vi "Begin.vi"(8 "error in":errorcluster) -> (0 "error out":errorcluster)   [LabVIEW 2019]
doc: "Called before other user functions, this VI is expected to open initial I/O refnums, load in file data, and do all program initialization. Notice that the <B>error out</B> terminal is simply used for data flow. Wiring it to other structures or subVIs ensures that this VI runs first."
uses:
  <vilib>/Rock Robotics/SystemInterfaces/i2clib/i2c_bus.ctl
  <vilib>/Rock Robotics/WPI/DriverStation/WPI_DriverStationRobotMode2.ctl
  <vilib>/Rock Robotics/WPI/Joystick/WPI_JoystickDeviceEnum.ctl
  <vilib>/Rock Robotics/WPI/SafetyOutput/WPI_SafetyOutputConfigMenu.ctl
  <vilib>/Rock Robotics/WPI/ThirdParty/Phoenix-LabVIEW/Motor Controller/Controls/CTRE_Phoenix_MotorControl_FeedbackDevice.ctl
  <vilib>/Rock Robotics/WPI/Solenoid/WPI_SolenoidChannel.ctl
  <vilib>/Rock Robotics/WPI/ThirdParty/Phoenix-LabVIEW/Motor Controller/Controls/CTRE_Phoenix_MotorControl_ControlMode.ctl
  <vilib>/Rock Robotics/WPI/ThirdParty/Phoenix-LabVIEW/Motor Controller/Controls/CTRE_Phoenix_MotorControl_FeedbackDevice_TalonFX.ctl
  <vilib>/Rock Robotics/WPI/ThirdParty/Phoenix-LabVIEW/Motor Controller/Controls/CTRE_Phoenix_MotorControl_NeutralMode.ctl
  <vilib>/Rock Robotics/WPI/ThirdParty/REV Robotics/SPARK MAX/Typedef/Spark MAX Motor Type.ctl
  <vilib>/Rock Robotics/WPI/ThirdParty/Phoenix-LabVIEW/Motor Controller/Controls/CTRE_Phoenix_MotorControl_VelocityMeasurementPeriod.ctl
  <vilib>/Rock Robotics/SystemInterfaces/DIO/FPGA_DIOChannel.ctl
  Robot Global Data.vi
  <vilib>/Rock Robotics/Network Tables/NT Write String Array.vi
  <vilib>/Rock Robotics/WPI/Solenoid/WPI_SolenoidOpenDouble.vi
  <vilib>/Rock Robotics/WPI/RobotDrive/WPI_RobotDriveOpen4MotorWithExistingMotors.vi
panel:
  in  "Blue Calibration":cluster{"R":dbl, "G":dbl, "B":dbl}={"R"=0.143, "G"=0.427, "B"=0.429}
  in  "Green Calibration":cluster{"R":dbl, "G":dbl, "B":dbl}={"R"=0.197, "G"=0.561, "B"=0.24}
  in  "Red Calibration":cluster{"R":dbl, "G":dbl, "B":dbl}={"R"=0.561, "G"=0.323, "B"=0.114}
  in  "Yellow Calibration":cluster{"R":dbl, "G":dbl, "B":dbl}={"R"=0.361, "G"=0.524, "B"=0.113}
  in  "I2C Bus":T1
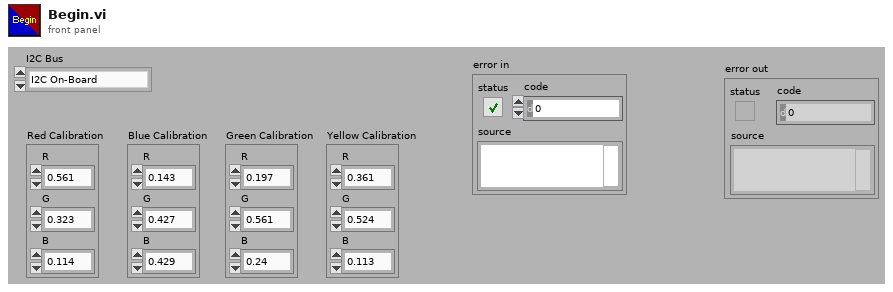
[diagram p1: front panel]
types:
  T1 = typedef "i2c_bus.ctl" = enum16{"I2C On-Board", "I2C MXP", "Invalid"}
  T2 = typedef "WPI_SolenoidChannel.ctl" = enum8{"Solenoid 0", "Solenoid 1", "Solenoid 2", "Solenoid 3", "Solenoid 4", "Solenoid 5", "Solenoid 6", "Solenoid 7", "Invalid"}
  T3 = typedef "FPGA_DIOChannel.ctl" = enum8{"DIO 0", "DIO 1", "DIO 2", "DIO 3", "DIO 4", "DIO 5", "DIO 6", "DIO 7", "DIO 8", "DIO 9", "DIO MXP 0", "DIO MXP 1", "DIO MXP 2", "DIO MXP 3", "DIO MXP 4", "DIO MXP 5", "DIO MXP 6", "DIO MXP 7", "DIO MXP 8", "DIO MXP 9", "DIO MXP 10", "DIO MXP 11", "DIO MXP 12", "DIO MXP 13", "DIO MXP 14", "DIO MXP 15", "SPI Port CS1", "SPI Port CS2", "SPI Port CS3", "SPI Port MISO", "SPI Port MOSI", "Invalid"}
  T4 = typedef "CTRE_Phoenix_MotorControl_VelocityMeasurementPeriod.ctl" = u16
  T5 = typedef "CTRE_Phoenix_MotorControl_NeutralMode.ctl" = enum8{"EEPROMSetting", "Override to Coast", "Override to Brake"}
  T6 = typedef "CTRE_Phoenix_MotorControl_FeedbackDevice_TalonFX.ctl" = i8
  T7 = typedef "CTRE_Phoenix_MotorControl_ControlMode.ctl" = u16
  T8 = typedef "Spark MAX Motor Type.ctl" = enum16{"Brushed", "Brushless"}
  T9 = typedef "CTRE_Phoenix_MotorControl_FeedbackDevice.ctl" = i8
  T10 = typedef "WPI_SafetyOutputConfigMenu.ctl" = enum16{"Enable", "Disable"}
  T11 = typedef "WPI_JoystickDeviceEnum.ctl" = enum16{"USB 0", "USB 1", "USB 2", "USB 3", "USB 4", "USB 5"}
  T12 = typedef "WPI_DriverStationRobotMode2.ctl" = enum16{"Autonomous Disabled", "Autonomous Enabled", "Teleop Disabled", "Teleop Enabled", "Disconnected", "Finish", "Test Disabled", "Test Enabled", "Emergency Stopped"}
  T13 = typedef "Color Sensor V3 DevRef.ctl" = cluster{"I2CDevRef":T14}
  T14 = typedef "WPI_I2CDevRef.ctl" = cluster{"DevStatus":errorcluster, "Device Address":u8, "Handle":i32, "I2C Bus":T1}
  T15 = typedef "WPI_JoystickDevRef.ctl" = cluster{"Device":T11}
  T16 = typedef "WPI_DigitalInputDevRef.ctl" = cluster{"DevStatus":errorcluster, "DIO Channel":T3}
  T17 = typedef "WPI_MotorControlDeviceRef.ctl" = cluster{"DeviceStatus":errorcluster, "Type":T18, "PWM":cluster{"PWM Channel":T19, "DeadBand":T20}, "CAN":cluster{"Device Number":u8, "SetOutput VI Ref":variant, "GetOutput VI Ref":variant, "Enable VI Ref":variant, "Disable VI Ref":variant, "Data":variant}, "Invert":bool, "DIO PWM":cluster{"PWM \"Enable\" Channel":T19, "DIOChannel":T3, "PWM Rate":dbl}}
  T18 = typedef "WPI_MotorControlType.ctl" = enum16{"PWM", "CAN", "DIO PWM"}
  T19 = typedef "FPGA_DIOPWMChannel.ctl" = enum8{"PWM 0", "PWM 1", "PWM 2", "PWM 3", "PWM 4", "PWM 5", "PWM 6", "PWM 7", "PWM 8", "PWM 9", "PWM MXP 0", "PWM MXP 1", "PWM MXP 2", "PWM MXP 3", "PWM MXP 4", "PWM MXP 5", "PWM MXP 6", "PWM MXP 7", "PWM MXP 8", "PWM MXP 9", "Invalid"}
  T20 = typedef "WPI_PWMDeadband.ctl" = cluster{"Name":string, "maxPositivePwm":i32, "minPositivePwm":i32, "centerPwm":i32, "maxNegativePwm":i32, "minNegativePwm":i32, "angularRange":u16}
  T21 = typedef "WPI_SolenoidDevRef.ctl" = cluster{"DevStatus":errorcluster, "Pneumatics Control Module":u8, "Forward Solenoid Channel":T2, "Reverse Solenoid Channel":T2}
  T22 = typedef "WPI_RobotDriveDevRef.ctl" = cluster{"DevStatus":errorcluster, "Motors[]":T17[], "Square Inputs":bool, "Max Output":dbl}
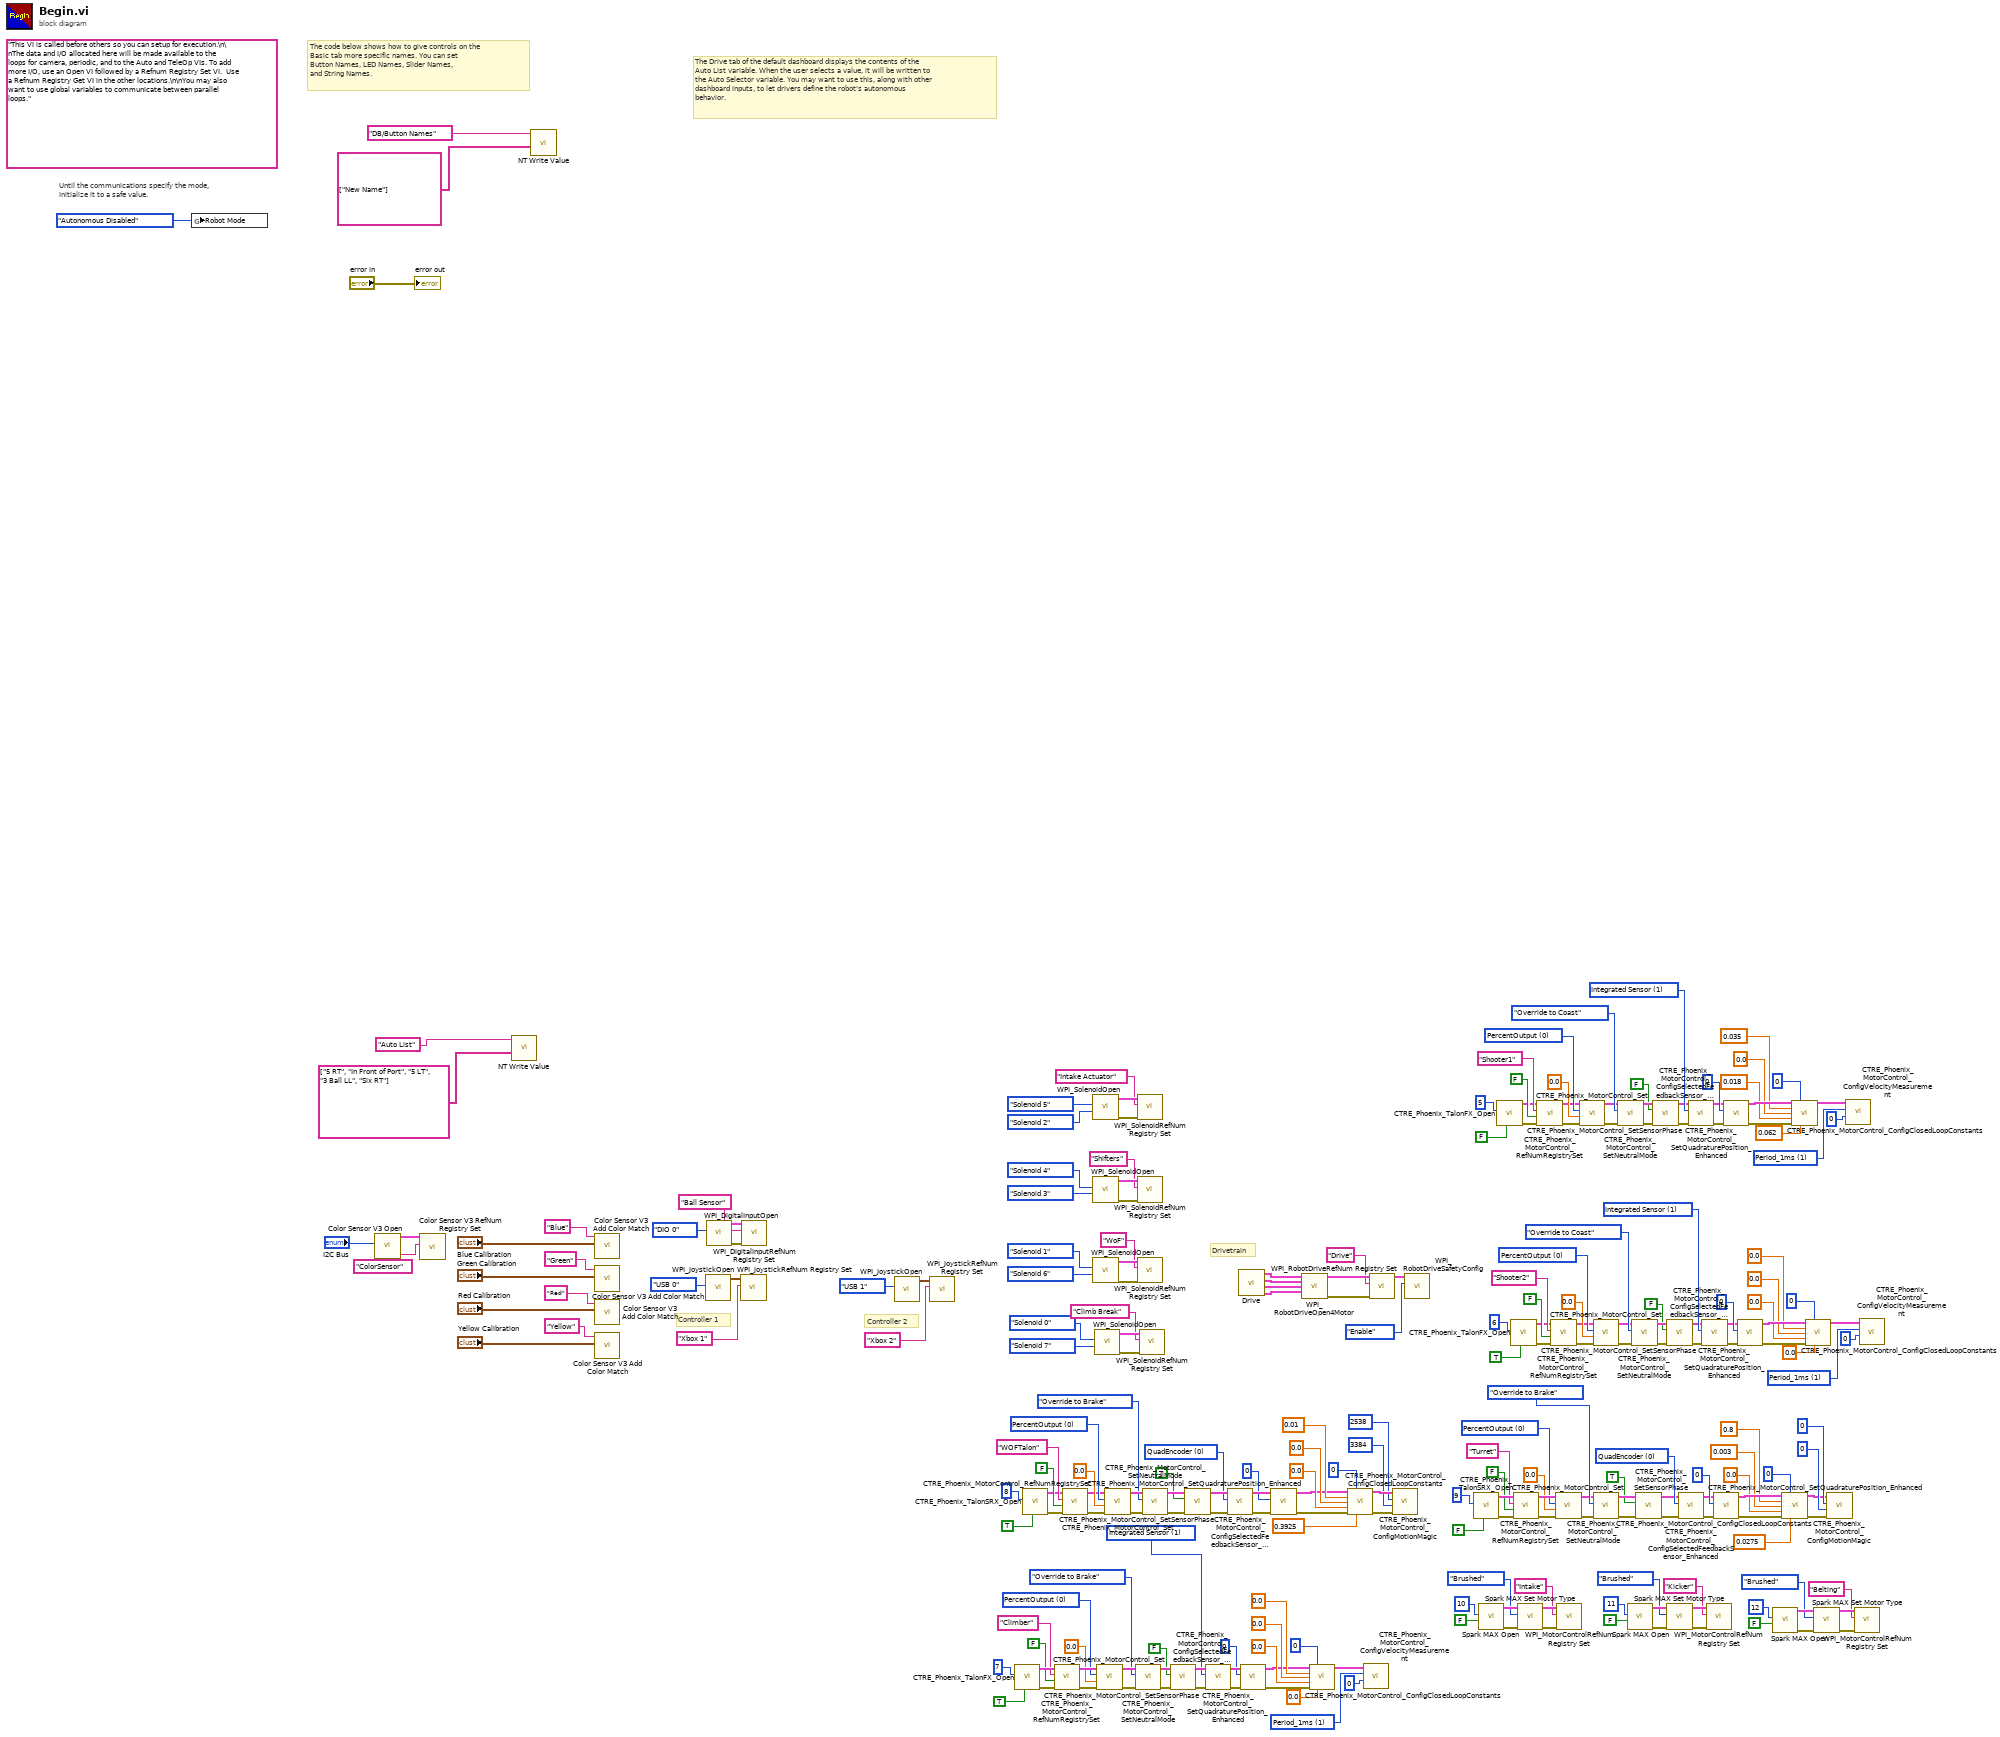
[diagram p0: block diagram]
diagram:
  w21 = T4 1 items=["Period_1ms"=1, "Period_2ms"=2, "Period_5ms"=5, "Period_10ms"=10, "Period_20ms"=20, "Period_25ms"=25, "Period_50ms"=50, "Period_100ms"=100] ("Velocity Measurement Period")
  w82 = T4 1 items=["Period_1ms"=1, "Period_2ms"=2, "Period_5ms"=5, "Period_10ms"=10, "Period_20ms"=20, "Period_25ms"=25, "Period_50ms"=50, "Period_100ms"=100] ("Velocity Measurement Period")
  w66 = T6 1 items=["Integrated Sensor"=1, "Sensor Sum (S0 + S1)"=9, "Sensor Difference (D0 - D1)"=10, "Remote Source 0"=11, "Remote Source 1"=12, "None"=14, "Software Emulated"=15] ("Talon FX Feedback Device")
  w64 = T7 0 items=["PercentOutput"=0, "Position"=1, "Velocity"=2, "Current"=3, "Follower"=5, "MotionProfile"=6, "MotionMagic"=7, "MotionProfileArc"=10, "Disabled"=15] ("Control Mode")
  w47 = T6 1 items=["Integrated Sensor"=1, "Sensor Sum (S0 + S1)"=9, "Sensor Difference (D0 - D1)"=10, "Remote Source 0"=11, "Remote Source 1"=12, "None"=14, "Software Emulated"=15] ("Talon FX Feedback Device")
  w45 = T7 0 items=["PercentOutput"=0, "Position"=1, "Velocity"=2, "Current"=3, "Follower"=5, "MotionProfile"=6, "MotionMagic"=7, "MotionProfileArc"=10, "Disabled"=15] ("Control Mode")
  w128 = T9 0 items=["None"=-1, "QuadEncoder"=0, "Analog"=2, "Tachometer"=4, "Pulse Width Encoded Position"=8, "Sensor Sum (S0 + S1)"=9, "Sensor Difference (D0 - D1)"=10, "Remote Source 0"=11, "Remote Source 1"=12, "Software Emulated"=15] ("Feedback Device")
  w123 = T7 0 items=["PercentOutput"=0, "Position"=1, "Velocity"=2, "Current"=3, "Follower"=5, "MotionProfile"=6, "MotionMagic"=7, "MotionMagicArc"=8, "MotionProfileArc"=10, "Disabled"=15] ("Control Mode")
  w143 = T4 1 items=["Period_1ms"=1, "Period_2ms"=2, "Period_5ms"=5, "Period_10ms"=10, "Period_20ms"=20, "Period_25ms"=25, "Period_50ms"=50, "Period_100ms"=100] ("Velocity Measurement Period")
  w155 = T6 1 items=["Integrated Sensor"=1, "Sensor Sum (S0 + S1)"=9, "Sensor Difference (D0 - D1)"=10, "Remote Source 0"=11, "Remote Source 1"=12, "None"=14, "Software Emulated"=15] ("Talon FX Feedback Device")
  w158 = T7 0 items=["PercentOutput"=0, "Position"=1, "Velocity"=2, "Current"=3, "Follower"=5, "MotionProfile"=6, "MotionMagic"=7, "MotionProfileArc"=10, "Disabled"=15] ("Control Mode")
  w196 = T9 0 items=["None"=-1, "QuadEncoder"=0, "Analog"=2, "Tachometer"=4, "Pulse Width Encoded Position"=8, "Sensor Sum (S0 + S1)"=9, "Sensor Difference (D0 - D1)"=10, "Remote Source 0"=11, "Remote Source 1"=12, "Software Emulated"=15] ("Feedback Device")
  w201 = T7 0 items=["PercentOutput"=0, "Position"=1, "Velocity"=2, "Current"=3, "Follower"=5, "MotionProfile"=6, "MotionMagic"=7, "MotionMagicArc"=8, "MotionProfileArc"=10, "Disabled"=15] ("Control Mode")
  (unwired) "This VI is called before others so you can setup for execution.\n\nThe data and I/O allocated here will be made available to the loops for camera, periodic, and to the Auto and TeleOp VIs. To add more I/O, use an Open VI followed by a Refnum Registry Set VI.  Use a Refnum Registry Get VI in the other locations.\n\nYou may also want to use global variables to communicate between parallel loops."
  # "Controller 2"
  # "Controller 1"
  # "Drivetrain"
  # "The Drive tab of the default dashboard displays the contents of the\nAuto List variable. When the user selects a value, it will be written to\nthe Auto Selector variable. You may want to use this, along with other\ndashboard inputs, to let drivers define the robot's autonomous\nbehavior."
  # "The code below shows how to give controls on the\nBasic tab more specific names. You can set\nButton Names, LED Names, Slider Names,\nand String Names."
  # "Until the communications specify the mode,\ninitialize it to a safe value."
  n1 = global write "Robot Global Data.vi" "Robot Mode"(WPI_DriverStationRobotMode2."Autonomous Disabled" ("Robot Mode")) -> ()
  n2 = call <vilib>:"Color Sensor V3 Open.vi"("I2C Bus"="I2C Bus") -> ("ColorSensorDevRef"=w224:T13)  [unwired: 9 in, 1 out]
  n3 = call <vilib>:"Color Sensor V3 RefNum Registry Set.vi"("refnum name"="ColorSensor", "ColorSensorDevRef"=w224) -> ()  [unwired: 8 in, 2 out]
  n4 = call-poly <vilib>:"NT Write Value.vi"("String Array"=string[] ["5 RT", "In Front of Port", "5 LT", "3 Ball LL", "Six RT"], "Name"="Auto List") -> ()  [unwired: 9 in, 1 out]
  n5 = call-poly <vilib>:"NT Write Value.vi"("String Array"=string[] ["New Name"], "Name"="DB/Button Names") -> ()  [unwired: 9 in, 1 out]
  n6 = call <vilib>:"Color Sensor V3 Add Color Match.vi"("Color"="Blue Calibration", "Name"="Blue") -> ()  [unwired: 10 in]
  n7 = call <vilib>:"Color Sensor V3 Add Color Match.vi"("Color"="Green Calibration", "Name"="Green") -> ()  [unwired: 10 in]
  n8 = call <vilib>:"Color Sensor V3 Add Color Match.vi"("Color"="Red Calibration", "Name"="Red") -> ()  [unwired: 10 in]
  n9 = call <vilib>:"Color Sensor V3 Add Color Match.vi"("Color"="Yellow Calibration", "Name"="Yellow") -> ()  [unwired: 10 in]
  n10 = call <vilib>:"WPI_JoystickOpen.vi"("JoystickDevice"=WPI_JoystickDeviceEnum."USB 0") -> ("JoystickDevRef"=w240:T15)  [unwired: 10 in]
  n11 = call <vilib>:"WPI_DigitalInputOpen.vi"("DIO Channel"=FPGA_DIOChannel."DIO 0") -> ("error out"=w20:errorcluster, "DigitalInputDevRef"=w19:T16)  [unwired: 9 in]
  n12 = call <vilib>:"WPI_JoystickRefNum Registry Set.vi"("refnum name"="Xbox 1", "JoystickDevRef"=w240) -> ()  [unwired: 8 in, 2 out]
  n13 = call <vilib>:"WPI_DigitalInputRefNum Registry Set.vi"("error in (no error)"=w20, "refnum name"="Ball Sensor", "DigitalInputDevRef"=w19) -> ()  [unwired: 7 in, 2 out]
  n14 = call <vilib>:"WPI_JoystickOpen.vi"("JoystickDevice"=WPI_JoystickDeviceEnum."USB 1") -> ("JoystickDevRef"=w221:T15)  [unwired: 10 in]
  n15 = call <vilib>:"WPI_JoystickRefNum Registry Set.vi"("refnum name"="Xbox 2", "JoystickDevRef"=w221) -> ()  [unwired: 8 in, 2 out]
  n16 = call <vilib>:"CTRE_Phoenix_TalonFX_Open.vi"("Invert"=TRUE, "Device Number"=u8 7) -> ("error out"=w173:errorcluster, "CAN Talon SRX Ref"=w172:T17)  [unwired: 8 in]
  n17 = call <vilib>:"CTRE_Phoenix_TalonSRX_Open.vi"("Invert"=TRUE, "Device Number"=u8 8) -> ("error out"=w137:errorcluster, "CAN Talon SRX Ref"=w138:T17)  [unwired: 8 in]
  n18 = call <vilib>:"CTRE_Phoenix_MotorControl_RefNumRegistrySet.vi"("error in (no error)"=w173, "Test Mode Only"=FALSE, "refnum name"="Climber", "PhoenixMotorControlDevRef"=w172) -> ("error out"=w171:errorcluster, "PhoenixMotorControlDevRef"=w170:T17)  [unwired: 6 in]
  n19 = call <vilib>:"CTRE_Phoenix_MotorControl_RefNumRegistrySet.vi"("error in (no error)"=w137, "Test Mode Only"=FALSE, "refnum name"="WOFTalon", "PhoenixMotorControlDevRef"=w138) -> ("error out"=w121:errorcluster, "PhoenixMotorControlDevRef"=w122:T17)  [unwired: 6 in]
  n20 = call-poly <vilib>:"WPI_SolenoidOpen.vi"("Reverse Solenoid Channel"=WPI_SolenoidChannel."Solenoid 2", "Forward Solenoid Channel"=WPI_SolenoidChannel."Solenoid 5") -> ("error out"=w7:errorcluster, "SolenoidDevRef"=w6:T21)  [unwired: 8 in]
  n21 = call-poly <vilib>:"WPI_SolenoidOpen.vi"("Reverse Solenoid Channel"=WPI_SolenoidChannel."Solenoid 3", "Forward Solenoid Channel"=WPI_SolenoidChannel."Solenoid 4") -> ("error out"=w177:errorcluster, "SolenoidDevRef"=w176:T21)  [unwired: 8 in]
  n22 = call-poly <vilib>:"WPI_SolenoidOpen.vi"("Reverse Solenoid Channel"=WPI_SolenoidChannel."Solenoid 6", "Forward Solenoid Channel"=WPI_SolenoidChannel."Solenoid 1") -> ("error out"=w16:errorcluster, "SolenoidDevRef"=w15:T21)  [unwired: 8 in]
  n23 = call-poly <vilib>:"WPI_SolenoidOpen.vi"("Reverse Solenoid Channel"=WPI_SolenoidChannel."Solenoid 7", "Forward Solenoid Channel"=WPI_SolenoidChannel."Solenoid 0") -> ("error out"=w12:errorcluster, "SolenoidDevRef"=w11:T21)  [unwired: 8 in]
  n24 = call <vilib>:"CTRE_Phoenix_MotorControl_Set.vi"("error in (no error)"=w171, "Output"=0.0, "Control Mode"=w158, "PhoenixMotorControlDevRef"=w170) -> ("error out"=w169:errorcluster, "PhoenixMotorControlDevRef"=w168:T17)  [unwired: 6 in]
  n25 = call <vilib>:"CTRE_Phoenix_MotorControl_Set.vi"("error in (no error)"=w121, "Output"=0.0, "Control Mode"=w123, "PhoenixMotorControlDevRef"=w122) -> ("error out"=w132:errorcluster, "PhoenixMotorControlDevRef"=w136:T17)  [unwired: 6 in]
  n26 = call <vilib>:"CTRE_Phoenix_MotorControl_SetNeutralMode.vi"("error in (no error)"=w169, "Motor Control Neutral Mode"=CTRE_Phoenix_MotorControl_NeutralMode."Override to Brake", "PhoenixMotorControlDevRef"=w168) -> ("error out"=w167:errorcluster, "PhoenixMotorControlDevRef"=w166:T17)  [unwired: 7 in]
  n27 = call <vilib>:"WPI_SolenoidRefNum Registry Set.vi"("error in (no error)"=w7, "refnum name"="Intake Actuator", "SolenoidDevRef"=w6) -> ()  [unwired: 7 in, 2 out]
  n28 = call <vilib>:"WPI_SolenoidRefNum Registry Set.vi"("error in (no error)"=w177, "refnum name"="Shifters", "SolenoidDevRef"=w176) -> ()  [unwired: 7 in, 2 out]
  n29 = call <vilib>:"WPI_SolenoidRefNum Registry Set.vi"("error in (no error)"=w16, "refnum name"="WoF", "SolenoidDevRef"=w15) -> ()  [unwired: 7 in, 2 out]
  n30 = call <vilib>:"WPI_SolenoidRefNum Registry Set.vi"("error in (no error)"=w12, "refnum name"="Climb Break", "SolenoidDevRef"=w11) -> ()  [unwired: 7 in, 2 out]
  n31 = call <vilib>:"CTRE_Phoenix_MotorControl_SetNeutralMode.vi"("error in (no error)"=w132, "Motor Control Neutral Mode"=CTRE_Phoenix_MotorControl_NeutralMode."Override to Brake", "PhoenixMotorControlDevRef"=w136) -> ("error out"=w134:errorcluster, "PhoenixMotorControlDevRef"=w133:T17)  [unwired: 7 in]
  n32 = call <vilib>:"CTRE_Phoenix_MotorControl_SetSensorPhase.vi"("error in (no error)"=w167, "PhaseSensor"=FALSE, "PhoenixMotorControlDevRef"=w166) -> ("error out"=w165:errorcluster, "PhoenixMotorControlDevRef"=w164:T17)  [unwired: 7 in]
  n33 = call <vilib>:"CTRE_Phoenix_MotorControl_SetSensorPhase.vi"("error in (no error)"=w134, "PhaseSensor"=TRUE, "PhoenixMotorControlDevRef"=w133) -> ("error out"=w130:errorcluster, "PhoenixMotorControlDevRef"=w129:T17)  [unwired: 7 in]
  n34 = call <vilib>:"CTRE_Phoenix_MotorControl_ConfigSelectedFeedbackSensor_TalonFX.vi"("error in (no error)"=w165, "Talon FX Feedback Device"=w155, "PhoenixMotorControlDevRef"=w164) -> ("error out"=w163:errorcluster, "PhoenixMotorControlDevRef"=w162:T17)  [unwired: 7 in]
  n35 = call <vilib>:"CTRE_Phoenix_MotorControl_ConfigSelectedFeedbackSensor_Enhanced.vi"("error in (no error)"=w130, "Feedback Device"=w128, "PhoenixMotorControlDevRef"=w129) -> ("error out"=w126:errorcluster, "PhoenixMotorControlDevRef"=w127:T17)  [unwired: 7 in]
  n36 = call "Drive.vi"() -> ("Front Right"=w178:T17, "Front Left"=w179:T17, "Rear Right"=w180:T17, "Rear Left"=w181:T17)  [unwired: 8 in]
  n37 = call <vilib>:"CTRE_Phoenix_MotorControl_SetQuadraturePosition_Enhanced.vi"("error in (no error)"=w163, "New Position"=0, "PhoenixMotorControlDevRef"=w162) -> ("error out"=w145:errorcluster, "PhoenixMotorControlDevRef"=w146:T17)  [unwired: 7 in]
  n38 = call <vilib>:"CTRE_Phoenix_MotorControl_SetQuadraturePosition_Enhanced.vi"("error in (no error)"=w126, "New Position"=0, "PhoenixMotorControlDevRef"=w127) -> ("error out"=w109:errorcluster, "PhoenixMotorControlDevRef"=w110:T17)  [unwired: 7 in]
  n39 = call-poly <vilib>:"WPI_RobotDriveOpen4Motor.vi"("Rear Left Motor Dev Ref"=w181, "Rear Right Motor Dev Ref"=w180, "Front Left Motor Dev Ref"=w179, "Front Right Motor Dev Ref"=w178) -> ("RobotDriveDevRef"=w219:T22, "error out"=w217:errorcluster)  [unwired: 10 in]
  n40 = call <vilib>:"CTRE_Phoenix_MotorControl_ConfigClosedLoopConstants.vi"("PhoenixMotorControlDevRef"=w146, "slotIdx"=0, "P"=0.0, "I"=0.0, "D"=0.0, "error in (no error)"=w145, "F"=0.0) -> ("PhoenixMotorControlDevRef"=w142:T17)  [unwired: 7 in, 1 out]
  n41 = call <vilib>:"CTRE_Phoenix_MotorControl_ConfigClosedLoopConstants.vi"("PhoenixMotorControlDevRef"=w110, "slotIdx"=0, "P"=0.01, "I"=0.0, "D"=0.0, "error in (no error)"=w109, "F"=0.3925) -> ("PhoenixMotorControlDevRef"=w118:T17, "error out"=w119:errorcluster)  [unwired: 7 in]
  n42 = call <vilib>:"CTRE_Phoenix_MotorControl_ConfigVelocityMeasurement.vi"("Window Size"=0, "Velocity Measurement Period"=w143, "PhoenixMotorControlDevRef"=w142) -> ()  [unwired: 7 in, 2 out]
  n43 = call <vilib>:"WPI_RobotDriveRefNum Registry Set.vi"("error in (no error)"=w217, "refnum name"="Drive", "RobotDriveDevRef"=w219) -> ("RobotDriveDevRef"=w216:T22)  [unwired: 1 in, 7 out]
  n44 = call <vilib>:"CTRE_Phoenix_MotorControl_ConfigMotionMagic.vi"("error in (no error)"=w119, "Acceleration"=3384, "Cruise Velocity"=2538, "PhoenixMotorControlDevRef"=w118) -> ()  [unwired: 6 in, 2 out]
  n45 = call <vilib>:"WPI_RobotDriveSafetyConfig.vi"("mode"=WPI_SafetyOutputConfigMenu."Enable", "RobotDriveDevRef"=w216) -> ()  [unwired: 8 in, 2 out]
  n46 = call <vilib>:"CTRE_Phoenix_TalonSRX_Open.vi"("Invert"=FALSE, "Device Number"=u8 9) -> ("error out"=w188:errorcluster, "CAN Talon SRX Ref"=w187:T17)  [unwired: 8 in]
  n47 = call <vilib>:"Spark MAX Open.vi"("Invert"=FALSE, "Device Number"=u8 10) -> ("error out"=w107:errorcluster, "MotorControlDeviceRef"=w108:T17)  [unwired: 8 in]
  n48 = call <vilib>:"CTRE_Phoenix_TalonFX_Open.vi"("Invert"=FALSE, "Device Number"=u8 5) -> ("error out"=w32:errorcluster, "CAN Talon SRX Ref"=w33:T17)  [unwired: 8 in]
  n49 = call <vilib>:"CTRE_Phoenix_TalonFX_Open.vi"("Invert"=TRUE, "Device Number"=u8 6) -> ("error out"=w51:errorcluster, "CAN Talon SRX Ref"=w52:T17)  [unwired: 8 in]
  n50 = call <vilib>:"CTRE_Phoenix_MotorControl_RefNumRegistrySet.vi"("error in (no error)"=w188, "Test Mode Only"=FALSE, "refnum name"="Turret", "PhoenixMotorControlDevRef"=w187) -> ("error out"=w203:errorcluster, "PhoenixMotorControlDevRef"=w202:T17)  [unwired: 6 in]
  n51 = call <vilib>:"Spark MAX Set Motor Type.vi"("error in (no error)"=w107, "Motor Type"=Spark_MAX_Motor_Type."Brushed", "MotorControlDevRef"=w108) -> ("error out"=w105:errorcluster, "MotorControlDeviceRef"=w104:T17)  [unwired: 7 in]
  n52 = call <vilib>:"CTRE_Phoenix_MotorControl_RefNumRegistrySet.vi"("error in (no error)"=w32, "Test Mode Only"=FALSE, "refnum name"="Shooter1", "PhoenixMotorControlDevRef"=w33) -> ("error out"=w34:errorcluster, "PhoenixMotorControlDevRef"=w35:T17)  [unwired: 6 in]
  n53 = call <vilib>:"CTRE_Phoenix_MotorControl_RefNumRegistrySet.vi"("error in (no error)"=w51, "Test Mode Only"=FALSE, "refnum name"="Shooter2", "PhoenixMotorControlDevRef"=w52) -> ("error out"=w53:errorcluster, "PhoenixMotorControlDevRef"=w54:T17)  [unwired: 6 in]
  n54 = call <vilib>:"CTRE_Phoenix_MotorControl_Set.vi"("error in (no error)"=w203, "Output"=0.0, "Control Mode"=w201, "PhoenixMotorControlDevRef"=w202) -> ("error out"=w193:errorcluster, "PhoenixMotorControlDevRef"=w189:T17)  [unwired: 6 in]
  n55 = call <vilib>:"WPI_MotorControlRefNum Registry Set.vi"("error in (no error)"=w105, "refnum name"="Intake", "MotorControlDevRef"=w104) -> ()  [unwired: 7 in, 2 out]
  n56 = call <vilib>:"CTRE_Phoenix_MotorControl_Set.vi"("error in (no error)"=w34, "Output"=0.0, "Control Mode"=w45, "PhoenixMotorControlDevRef"=w35) -> ("error out"=w36:errorcluster, "PhoenixMotorControlDevRef"=w37:T17)  [unwired: 6 in]
  n57 = call <vilib>:"CTRE_Phoenix_MotorControl_Set.vi"("error in (no error)"=w53, "Output"=0.0, "Control Mode"=w64, "PhoenixMotorControlDevRef"=w54) -> ("error out"=w55:errorcluster, "PhoenixMotorControlDevRef"=w56:T17)  [unwired: 6 in]
  n58 = call <vilib>:"CTRE_Phoenix_MotorControl_SetNeutralMode.vi"("error in (no error)"=w193, "Motor Control Neutral Mode"=CTRE_Phoenix_MotorControl_NeutralMode."Override to Brake", "PhoenixMotorControlDevRef"=w189) -> ("error out"=w191:errorcluster, "PhoenixMotorControlDevRef"=w192:T17)  [unwired: 7 in]
  n59 = call <vilib>:"CTRE_Phoenix_MotorControl_SetNeutralMode.vi"("error in (no error)"=w36, "Motor Control Neutral Mode"=CTRE_Phoenix_MotorControl_NeutralMode."Override to Coast", "PhoenixMotorControlDevRef"=w37) -> ("error out"=w38:errorcluster, "PhoenixMotorControlDevRef"=w39:T17)  [unwired: 7 in]
  n60 = call <vilib>:"Spark MAX Open.vi"("Invert"=FALSE, "Device Number"=u8 11) -> ("error out"=w91:errorcluster, "MotorControlDeviceRef"=w92:T17)  [unwired: 8 in]
  n61 = call <vilib>:"CTRE_Phoenix_MotorControl_SetNeutralMode.vi"("error in (no error)"=w55, "Motor Control Neutral Mode"=CTRE_Phoenix_MotorControl_NeutralMode."Override to Coast", "PhoenixMotorControlDevRef"=w56) -> ("error out"=w57:errorcluster, "PhoenixMotorControlDevRef"=w58:T17)  [unwired: 7 in]
  n62 = call <vilib>:"CTRE_Phoenix_MotorControl_SetSensorPhase.vi"("error in (no error)"=w191, "PhaseSensor"=TRUE, "PhoenixMotorControlDevRef"=w192) -> ("error out"=w194:errorcluster, "PhoenixMotorControlDevRef"=w195:T17)  [unwired: 7 in]
  n63 = call <vilib>:"CTRE_Phoenix_MotorControl_SetSensorPhase.vi"("error in (no error)"=w38, "PhaseSensor"=FALSE, "PhoenixMotorControlDevRef"=w39) -> ("error out"=w40:errorcluster, "PhoenixMotorControlDevRef"=w41:T17)  [unwired: 7 in]
  n64 = call <vilib>:"CTRE_Phoenix_MotorControl_SetSensorPhase.vi"("error in (no error)"=w57, "PhaseSensor"=FALSE, "PhoenixMotorControlDevRef"=w58) -> ("error out"=w59:errorcluster, "PhoenixMotorControlDevRef"=w60:T17)  [unwired: 7 in]
  n65 = call <vilib>:"Spark MAX Set Motor Type.vi"("error in (no error)"=w91, "Motor Type"=Spark_MAX_Motor_Type."Brushed", "MotorControlDevRef"=w92) -> ("error out"=w89:errorcluster, "MotorControlDeviceRef"=w88:T17)  [unwired: 7 in]
  n66 = call <vilib>:"CTRE_Phoenix_MotorControl_ConfigSelectedFeedbackSensor_Enhanced.vi"("error in (no error)"=w194, "Feedback Device"=w196, "PhoenixMotorControlDevRef"=w195) -> ("error out"=w198:errorcluster, "PhoenixMotorControlDevRef"=w197:T17)  [unwired: 7 in]
  n67 = call <vilib>:"CTRE_Phoenix_MotorControl_ConfigSelectedFeedbackSensor_TalonFX.vi"("error in (no error)"=w40, "Talon FX Feedback Device"=w47, "PhoenixMotorControlDevRef"=w41) -> ("error out"=w42:errorcluster, "PhoenixMotorControlDevRef"=w43:T17)  [unwired: 7 in]
  n68 = call <vilib>:"CTRE_Phoenix_MotorControl_ConfigSelectedFeedbackSensor_TalonFX.vi"("error in (no error)"=w59, "Talon FX Feedback Device"=w66, "PhoenixMotorControlDevRef"=w60) -> ("error out"=w61:errorcluster, "PhoenixMotorControlDevRef"=w62:T17)  [unwired: 7 in]
  n69 = call <vilib>:"WPI_MotorControlRefNum Registry Set.vi"("error in (no error)"=w89, "refnum name"="Kicker", "MotorControlDevRef"=w88) -> ()  [unwired: 7 in, 2 out]
  n70 = call <vilib>:"CTRE_Phoenix_MotorControl_SetQuadraturePosition_Enhanced.vi"("error in (no error)"=w198, "New Position"=0, "PhoenixMotorControlDevRef"=w197) -> ("error out"=w214:errorcluster, "PhoenixMotorControlDevRef"=w213:T17)  [unwired: 7 in]
  n71 = call <vilib>:"CTRE_Phoenix_MotorControl_SetQuadraturePosition_Enhanced.vi"("error in (no error)"=w42, "New Position"=0, "PhoenixMotorControlDevRef"=w43) -> ("error out"=w75:errorcluster, "PhoenixMotorControlDevRef"=w74:T17)  [unwired: 7 in]
  n72 = call <vilib>:"CTRE_Phoenix_MotorControl_SetQuadraturePosition_Enhanced.vi"("error in (no error)"=w61, "New Position"=0, "PhoenixMotorControlDevRef"=w62) -> ("error out"=w81:errorcluster, "PhoenixMotorControlDevRef"=w80:T17)  [unwired: 7 in]
  n73 = call <vilib>:"Spark MAX Open.vi"("Invert"=FALSE, "Device Number"=u8 12) -> ("error out"=w99:errorcluster, "MotorControlDeviceRef"=w100:T17)  [unwired: 8 in]
  n74 = call <vilib>:"CTRE_Phoenix_MotorControl_ConfigClosedLoopConstants.vi"("PhoenixMotorControlDevRef"=w213, "slotIdx"=0, "P"=0.8, "I"=0.003, "D"=0.0, "error in (no error)"=w214, "F"=0.0275) -> ("PhoenixMotorControlDevRef"=w205:T17, "error out"=w204:errorcluster)  [unwired: 7 in]
  n75 = call <vilib>:"CTRE_Phoenix_MotorControl_ConfigClosedLoopConstants.vi"("PhoenixMotorControlDevRef"=w74, "slotIdx"=0, "P"=0.035, "I"=0.0, "D"=0.018, "error in (no error)"=w75, "F"=0.062) -> ("PhoenixMotorControlDevRef"=w84:T17)  [unwired: 7 in, 1 out]
  n76 = call <vilib>:"CTRE_Phoenix_MotorControl_ConfigClosedLoopConstants.vi"("PhoenixMotorControlDevRef"=w80, "slotIdx"=0, "P"=0.0, "I"=0.0, "D"=0.0, "error in (no error)"=w81, "F"=0.0) -> ("PhoenixMotorControlDevRef"=w83:T17)  [unwired: 7 in, 1 out]
  n77 = call <vilib>:"Spark MAX Set Motor Type.vi"("error in (no error)"=w99, "Motor Type"=Spark_MAX_Motor_Type."Brushed", "MotorControlDevRef"=w100) -> ("error out"=w97:errorcluster, "MotorControlDeviceRef"=w96:T17)  [unwired: 7 in]
  n78 = call <vilib>:"CTRE_Phoenix_MotorControl_ConfigMotionMagic.vi"("error in (no error)"=w204, "Acceleration"=0, "Cruise Velocity"=0, "PhoenixMotorControlDevRef"=w205) -> ()  [unwired: 6 in, 2 out]
  n79 = call <vilib>:"CTRE_Phoenix_MotorControl_ConfigVelocityMeasurement.vi"("Window Size"=0, "Velocity Measurement Period"=w82, "PhoenixMotorControlDevRef"=w84) -> ()  [unwired: 7 in, 2 out]
  n80 = call <vilib>:"WPI_MotorControlRefNum Registry Set.vi"("error in (no error)"=w97, "refnum name"="Belting", "MotorControlDevRef"=w96) -> ()  [unwired: 7 in, 2 out]
  n81 = call <vilib>:"CTRE_Phoenix_MotorControl_ConfigVelocityMeasurement.vi"("Window Size"=0, "Velocity Measurement Period"=w21, "PhoenixMotorControlDevRef"=w83) -> ()  [unwired: 7 in, 2 out]
  "error out" <- "error in"
